vi "Oscilloscope.vi"() -> ()   [LabVIEW 2012]
uses:
  <vilib>/DAQmx/read.llb/DAQmx Read (Analog 1D Wfm NChan NSamp).vi
  <vilib>/DAQmx/create/channels.llb/DAQmx Create Channel (AI-Voltage-Basic).vi
  <vilib>/DAQmx/configure/timing.llb/DAQmx Timing (Sample Clock).vi
  <vilib>/DAQmx/miscellaneous.llb/DAQmx Fill In Error Info.vi
panel:
  in  "Physical Channel":tag="Dev1/ai0"
  in  "Time Window (s)":dbl=2.0
  in  "Frequency (MHz)":dbl=1.25 min=0.0 max=1.25 step=0.001
  out "amplitude":dbl
  out "reference":dbl
  out "Min voltage":dbl
  out "Max voltage":dbl
  out "Waveform Graph":waveform(dbl)[](graph)
  in  "stop (F)":bool
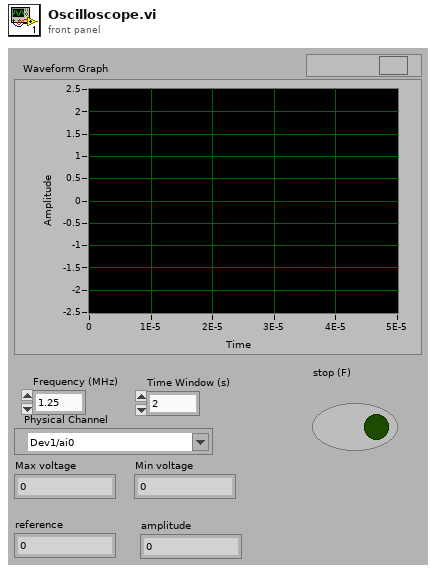
[diagram p1: front panel]
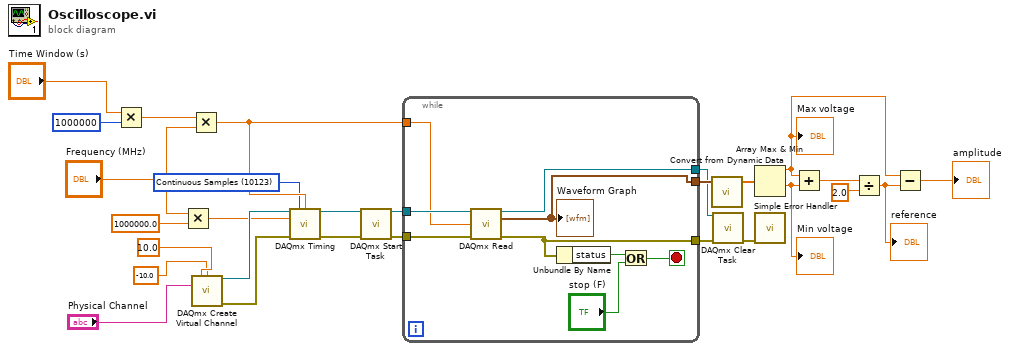
[diagram p0: block diagram]
diagram:
  w1 = 10123 items=["Finite Samples"=10178, "Continuous Samples"=10123, "Hardware Timed Single Point"=12522] ("sample mode")
  n1 = Multiply(x="Time Window (s)", y=1000000) -> (x*y=w11:dbl)
  n2 = Multiply(x="Frequency (MHz)", y=1000000.0) -> (x*y=w10:dbl)
  n3 = Multiply(x=w11, y="Frequency (MHz)") -> (x*y=w9:dbl)
  n4 = call-poly <vilib>:"DAQmx Create Virtual Channel.vi"("maximum value"=10.0, "minimum value"=-10.0, "physical channels"="Physical Channel") -> ("task out"=w20:refnum<k21>, "error out"=w19:errorcluster)  [unwired: 11 in]
  n5 = call-poly <vilib>:"DAQmx Timing.vi"("task/channels in"=w20, "sample mode"=w1, "samples per channel"=w9, "rate"=w10, "error in"=w19) -> ("task out"=w17:refnum<k21>, "error out"=w18:errorcluster)  [unwired: 9 in]
  n6 = call <vilib>:"DAQmx Start Task.vi"("task/channels in"=w17, "error in"=w18) -> ("task out"=w15:refnum<k21>, "error out"=w14:errorcluster)  [unwired: 12 in]
  n7 = while {
    tunnel: [w35] -> w28
    tunnel: w15 -> [w37]
    tunnel: w14 -> [w36]
    tunnel: w9 -> [w34]
    tunnel: [w33] -> w5
    tunnel: [w32] -> w4
    stop <- w30 stop-if-true
    n8 = call-poly <vilib>:"DAQmx Read.vi"("task/channels in"=w37, "number of samples per channel"=w34, "error in"=w36) -> ("task out"=w33:refnum<k21>, "data"=w35:waveform(dbl)[], "error out"=w32:errorcluster)  [unwired: 10 in]
    "Waveform Graph" <- w35
    n9 = Unbundle By Name(w32) -> ("status"=w31:bool)
    n10 = Or(x=w31, y="stop (F)") -> (x .or. y?=w30:bool)
  }
  n11 = call "Convert from Dynamic Data"("Dynamic Data Type"=w28) -> ("Array"=w27:dbl[])  [unwired: 3 in]
  n12 = call <vilib>:"DAQmx Clear Task.vi"("task in"=w5, "error in"=w4) -> ("error out"=w6:errorcluster)  [unwired: 13 in]
  n13 = Array Max & Min(array=w27) -> (max value=w23:dbl, min value=w26:dbl)  [unwired: 2 out]
  "Max voltage" <- w23
  "Min voltage" <- w26
  n14 = call <vilib>:"Simple Error Handler.vi"("error in (no error)"=w6) -> ()  [unwired: 4 in, 5 out]
  n15 = Add(x=w23, y=w26) -> (x+y=w25:dbl)
  n16 = Divide(x=w25, y=2.0) -> (x/y=w22:dbl)
  "reference" <- w22
  n17 = Subtract(x=w23, y=w22) -> (x-y=→"amplitude":dbl)
